vi "Startup.vi"(8 "error in (no error)":errorcluster, 11 "VolatusCore in":refnum<class "VolatusCore.lvclass">) -> (0 "error out":errorcluster, 3 "VolatusCore out":refnum<class "VolatusCore.lvclass">)   [LabVIEW 2020, in "Volatus.lvlib" / "VolatusCore.lvclass"]
uses:
  VolatusCore.lvclass
  C:/Program Files (x86)/National Instruments/LabVIEW 2020/vi.lib/ActorFramework/Actor/Actor.lvclass
  <vilib>/ActorFramework/Actor/Actor.lvclass/Actor.ctl
  <vilib>/ActorFramework/Message Enqueuer/Message Enqueuer.lvclass/Message Enqueuer.ctl
  <vilib>/ActorFramework/Message Enqueuer/Init from Existing Queue.vi
  <vilib>/ActorFramework/Message Enqueuer/Enqueue.vi
  VolatusCore Messages/Start Core Msg/Start Core Msg.lvclass
  C:/Program Files (x86)/National Instruments/LabVIEW 2020/vi.lib/ActorFramework/Message/Message.lvclass
  <vilib>/ActorFramework/Message Priority Queue/Priority Enqueue.vi
  <vilib>/ActorFramework/Message Enqueuer/Message Enqueuer.lvclass
  VolatusCore.lvclass/VolatusCore.ctl
  <vilib>/ActorFramework/Actor/Actor.lvclass
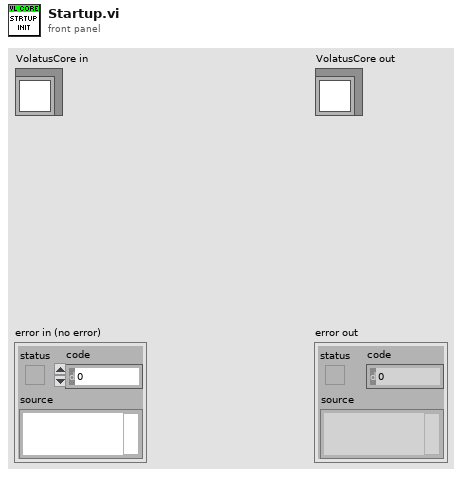
[diagram p1: front panel]
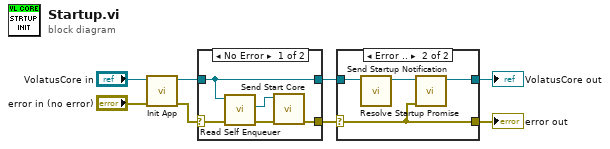
[diagram p0: block diagram]
diagram:
  n1 = call "Init App.vi"("error in (no error)"="error in (no error)", "VolatusCore in"="VolatusCore in") -> ("error out"=w6:errorcluster, "VolatusCore out"=w5:refnum<class "VolatusCore.lvclass">)  [unwired: 8 in]
  n2 = case shown="No Error" w6 {
    selector: w6 -> [w11 w14]
    tunnel: w5 -> [w9 w13]
    tunnel: [w10 w14] -> w2
    tunnel: [w9 w13] -> w4
    frame No Error {
      n3 = call <vilib>:"Read Self Enqueuer.vi"("Actor"=w9) -> ("Self Enqueuer"=w12:refnum<class "Message Enqueuer.lvclass">)  [unwired: 10 in]
      n4 = call "Send Start Core.vi"("error in (no error)"=w11, "Message Enqueuer"=w12) -> ("error out"=w10:errorcluster)  [unwired: 8 in, 1 out]
    }
    frame Error {
    }
  }
  n5 = case shown="Error .." w2 {
    selector: w2 -> [w15 w17]
    tunnel: [w15 w17] -> w1
    tunnel: [w16 w18] -> w3
    tunnel: w4 -> [w16 w19]
    frame No Error {
    }
    frame Error {
      n6 = call "Resolve Startup Promise.vi"("VolatusCore in"=w19) -> ("VolatusCore out"=w20:refnum<class "VolatusCore.lvclass">)  [unwired: 9 in, 1 out]
      n7 = call "Send Startup Notification.vi"("error in (no error)"=w17, "VolatusCore in"=w20) -> ("VolatusCore out"=w18:refnum<class "VolatusCore.lvclass">)  [unwired: 8 in, 1 out]
    }
  }
  "error out" <- w1
  "VolatusCore out" <- w3
